vi "TDMS_Open.vi"(8 "错误输入":errorcluster, 10 "文件路径":path=path "C:/Users/Administrator/Desktop/LabVIEW National Game Prj/KnockOut_R2/Solution/MySolution/LargeWf.tdms") -> (0 "错误输出":errorcluster, 1 "通道":string[](array[string]), 2 "组名称":string, 3 "tdms文件输出":refnum<k34>)   [LabVIEW 2011]
doc: "打开TDMS文件, 并传出TDMS文件的信息."
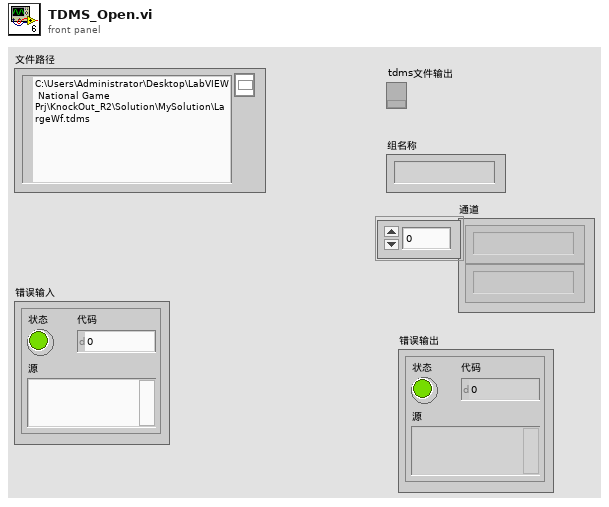
[diagram p1: front panel]
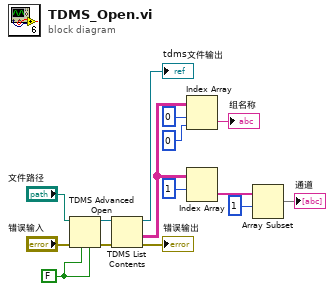
[diagram p0: block diagram]
diagram:
  w14 = FALSE ("禁用缓冲？(T)")
  n1 = TDMS Advanced Open(4:w14, 6:w14, 8:"错误输入", 11:"文件路径") -> (0:w10:errorcluster, 3:w13:refnum<k34>)  [unwired: 1 in, 1 out]
  n2 = TDMS List Contents(4:w10, 7:w13) -> (0:→"错误输出":errorcluster, 1:w5:string[][], 3:→"tdms文件输出":refnum<k34>)  [unwired: 1 in, 1 out]
  n3 = Index Array(array=w5, index (row)=0 ("索引 (行)"), index (col)=0 ("禁用的索引 (列)")) -> (element=→"组名称":string)
  n4 = Index Array(array=w5, index (row)=1 ("索引 (行)")) -> (element=w3:string[])  [unwired: 1 in]
  n5 = Array Subset(array=w3, index=1 ("索引")) -> (→"通道":string[])  [unwired: 1 in]
